vi "TEST_Python.vi"() -> ()   [LabVIEW 2021]
panel:
  out "Array":dbl[](array[numeric])
  in  "function name":string
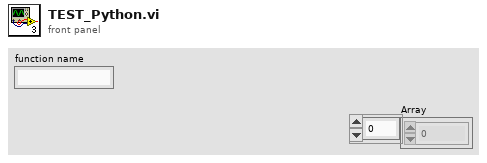
[diagram p1: front panel]
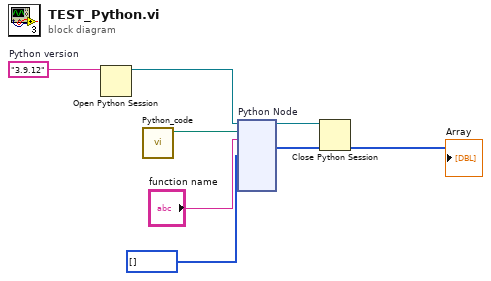
[diagram p0: block diagram]
diagram:
  w7 = "3.9.12"  # Python version
  n1 = Open Python Session(python version=w7) -> (session out=w6:refnum<k35>)  [unwired: 2 in, 1 out]
  n2 = call "Python_code.vi"() -> ("appended path"=w4:path)  [unwired: 11 in]
  n3 = node "Python Node"(w6, w4, "function name", i32[] []) -> (w5:refnum<k35>, →"Array":i32[])  [unwired: 9 in, 3 out]
  n4 = Close Python Session(session in=w5) -> ()  [unwired: 1 in, 1 out]
